vi "Lancing Math Algo.vi"(0 "Wm":dbl format="%#_13g", 1 "Curl Gap":dbl format="%#_13g", 5 "Hm":dbl format="%#_13g", 7 "sin_net":dbl format="%#_13g", 9 "cos_net":dbl format="%#_13g", 11 "Hm'":dbl) -> (4 "Lancing":dbl)   [LabVIEW 2015]
panel:
  out "H":dbl
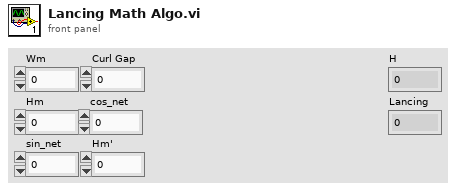
[diagram p1: front panel]
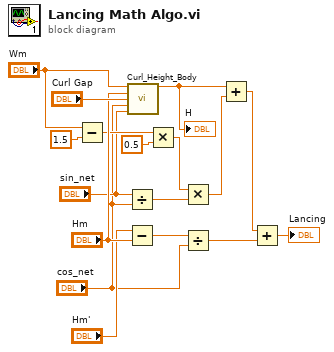
[diagram p0: block diagram]
diagram:
  n1 = Subtract(x="Wm", y=1.5) -> (x-y=w8:dbl)
  n2 = Divide(x="sin_net", y="cos_net") -> (x/y=w15:dbl)
  n3 = Subtract(x="Hm'", y="Hm") -> (x-y=w4:dbl)
  n4 = call "Curl_Height_Body.vi"("Wm"="Wm", "Hm"="Hm", "Curl Gap"="Curl Gap", "cos_net"="cos_net", "sin_net"="sin_net") -> ("H"=w5:dbl)  [unwired: 10 in]
  "H" <- w5
  n5 = Multiply(x=w8, y=0.5) -> (x*y=w6:dbl)
  n6 = Multiply(x=w6, y=w15) -> (x*y=w13:dbl)
  n7 = Divide(x=w4, y="cos_net") -> (x/y=w3:dbl)
  n8 = Add(x=w5, y=w13) -> (x+y=w12:dbl)
  n9 = Add(x=w12, y=w3) -> (x+y=→"Lancing":dbl)
